vi "メイン.vi"() -> (2 "測定周期/ms":dbl, 3 "値転記用配列":T2[](array[typedef]))   [LabVIEW 2021] (continued)
              n6483 = property on="メイン測定ボタン_連続 4" class="Bool (指定)"("DisabledEnum"=w8451) -> ()  [unwired: 2 in, 2 out]
            }
            frame 4 {
              n6484 = property on="メイン測定ボタン_単発 5" class="Bool (指定)"("DisabledEnum"=w8452) -> ()  [unwired: 2 in, 2 out]
              n6485 = property on="メイン測定ボタン_連続 5" class="Bool (指定)"("DisabledEnum"=w8452) -> ()  [unwired: 2 in, 2 out]
            }
            frame 5 {
              n6486 = property on="メイン測定ボタン_連続 6" class="Bool (指定)"("DisabledEnum"=w8453) -> ()  [unwired: 2 in, 2 out]
              n6487 = property on="メイン測定ボタン_単発 6" class="Bool (指定)"("DisabledEnum"=w8453) -> ()  [unwired: 2 in, 2 out]
            }
            frame 6 {
              n6488 = property on="メイン測定ボタン_連続 7" class="Bool (指定)"("DisabledEnum"=w8454) -> ()  [unwired: 2 in, 2 out]
              n6489 = property on="メイン測定ボタン_単発 7" class="Bool (指定)"("DisabledEnum"=w8454) -> ()  [unwired: 2 in, 2 out]
            }
            frame 7 {
              n6490 = property on="メイン測定ボタン_単発 8" class="Bool (指定)"("DisabledEnum"=w8455) -> ()  [unwired: 2 in, 2 out]
              n6491 = property on="メイン測定ボタン_連続 8" class="Bool (指定)"("DisabledEnum"=w8455) -> ()  [unwired: 2 in, 2 out]
            }
            frame 8 {
              n6492 = property on="メイン測定ボタン_単発 9" class="Bool (指定)"("DisabledEnum"=w8456) -> ()  [unwired: 2 in, 2 out]
              n6493 = property on="メイン測定ボタン_連続 9" class="Bool (指定)"("DisabledEnum"=w8456) -> ()  [unwired: 2 in, 2 out]
            }
            frame 9 {
              n6494 = property on="メイン測定ボタン_単発 10" class="Bool (指定)"("DisabledEnum"=w8457) -> ()  [unwired: 2 in, 2 out]
              n6495 = property on="メイン測定ボタン_連続 10" class="Bool (指定)"("DisabledEnum"=w8457) -> ()  [unwired: 2 in, 2 out]
            }
            frame 10 {
              n6496 = property on="メイン測定ボタン_単発 11" class="Bool (指定)"("DisabledEnum"=w8458) -> ()  [unwired: 2 in, 2 out]
              n6497 = property on="メイン測定ボタン_連続 11" class="Bool (指定)"("DisabledEnum"=w8458) -> ()  [unwired: 2 in, 2 out]
            }
            frame 11 {
              n6498 = property on="メイン測定ボタン_連続 12" class="Bool (指定)"("DisabledEnum"=w8459) -> ()  [unwired: 2 in, 2 out]
              n6499 = property on="メイン測定ボタン_単発 12" class="Bool (指定)"("DisabledEnum"=w8459) -> ()  [unwired: 2 in, 2 out]
            }
          }
        }
        n6500 = property on="TOPページへ" class="Bool"("DisabledEnum"=w8433) -> ()  [unwired: 2 in, 2 out]
        n6501 = property on="保存して終了" class="Bool"("DisabledEnum"=w8433) -> ()  [unwired: 2 in, 2 out]
        n6502 = property on="保存せずに" class="Bool"("DisabledEnum"=w8433) -> ()  [unwired: 2 in, 2 out]
      }
      event Value Change {
        n6503 = event-data() -> ()  [unwired: 1 in, 1 out]
        n6504 = Enqueue Element(queue=w8543, element="ON/OFF1", error in (no error)=w8542) -> ()  [unwired: 1 in, 3 out]
      }
      event Value Change {
        n6505 = event-data() -> ()  [unwired: 1 in, 1 out]
        n6506 = Enqueue Element(queue=w8546, element="ON/OFF2", error in (no error)=w8545) -> ()  [unwired: 1 in, 3 out]
      }
      event Value Change {
        n6507 = event-data() -> ()  [unwired: 1 in, 6 out]
        n6508 = Enqueue Element(queue=w8549, element="ON/OFF3", error in (no error)=w8548) -> ()  [unwired: 1 in, 3 out]
      }
      event Value Change {
        n6509 = event-data() -> ()  [unwired: 1 in, 6 out]
        n6510 = Enqueue Element(queue=w8552, element="ON/OFF4", error in (no error)=w8551) -> ()  [unwired: 1 in, 3 out]
      }
      event Value Change {
        n6511 = event-data() -> ()  [unwired: 1 in, 6 out]
        n6512 = Enqueue Element(queue=w8555, element="ON/OFF5", error in (no error)=w8554) -> ()  [unwired: 1 in, 3 out]
      }
      event Value Change {
        n6513 = event-data() -> ()  [unwired: 1 in, 6 out]
        n6514 = Enqueue Element(queue=w8558, element="ON/OFF6", error in (no error)=w8557) -> ()  [unwired: 1 in, 3 out]
      }
      event Value Change {
        n6515 = event-data() -> ()  [unwired: 1 in, 6 out]
        n6516 = Enqueue Element(queue=w8561, element="ON/OFF7", error in (no error)=w8560) -> ()  [unwired: 1 in, 3 out]
      }
      event Value Change {
        n6517 = event-data() -> ()  [unwired: 1 in, 6 out]
        n6518 = Enqueue Element(queue=w8564, element="ON/OFF8", error in (no error)=w8563) -> ()  [unwired: 1 in, 3 out]
      }
      event Value Change {
        n6519 = event-data() -> ()  [unwired: 1 in, 6 out]
        n6520 = Enqueue Element(queue=w8567, element="ON/OFF9", error in (no error)=w8566) -> ()  [unwired: 1 in, 3 out]
      }
      event Value Change {
        n6521 = event-data() -> ()  [unwired: 1 in, 6 out]
        n6522 = Enqueue Element(queue=w8570, element="ON/OFF10", error in (no error)=w8569) -> ()  [unwired: 1 in, 3 out]
      }
      event Value Change {
        n6523 = event-data() -> ()  [unwired: 1 in, 6 out]
        n6524 = Enqueue Element(queue=w8573, element="ON/OFF11", error in (no error)=w8572) -> ()  [unwired: 1 in, 3 out]
      }
      event Value Change {
        n6525 = event-data() -> ()  [unwired: 1 in, 6 out]
        n6526 = Enqueue Element(queue=w8576, element="ON/OFF12", error in (no error)=w8575) -> ()  [unwired: 1 in, 3 out]
      }
    }
  }
  n6527 = while {
    i -> [w8578]
    stop <- w8579 stop-if-true
    n6528 = case shown="0, デフォルト" w8578 {
      tunnel: [TRUE _] -> w8579
      frame 1 {
      }
      frame 0, Default {
        n6529 = while {
          stop <- w8581 stop-if-true
          n6530 = flat-sequence {
            tunnel: [TRUE] -> w8581
            frame #0 {
            }
          }
        }
      }
    }
  }
  n6531 = Release Queue(queue=w9, error in (no error)=w8) -> (error out=→"キューエラー出力":errorcluster)  [unwired: 1 in, 2 out]
